vi "Analysis.vi"() -> ()   [LabVIEW 2015, in "SubVIs.lvlib"]
uses:
  SubVIs.lvlib
panel:
  out "SPL":dynamicdata(graph)
  out "Audio":dynamicdata(graph)
  out "Pressure":dynamicdata(graph)
  out "Flow":dynamicdata(graph)
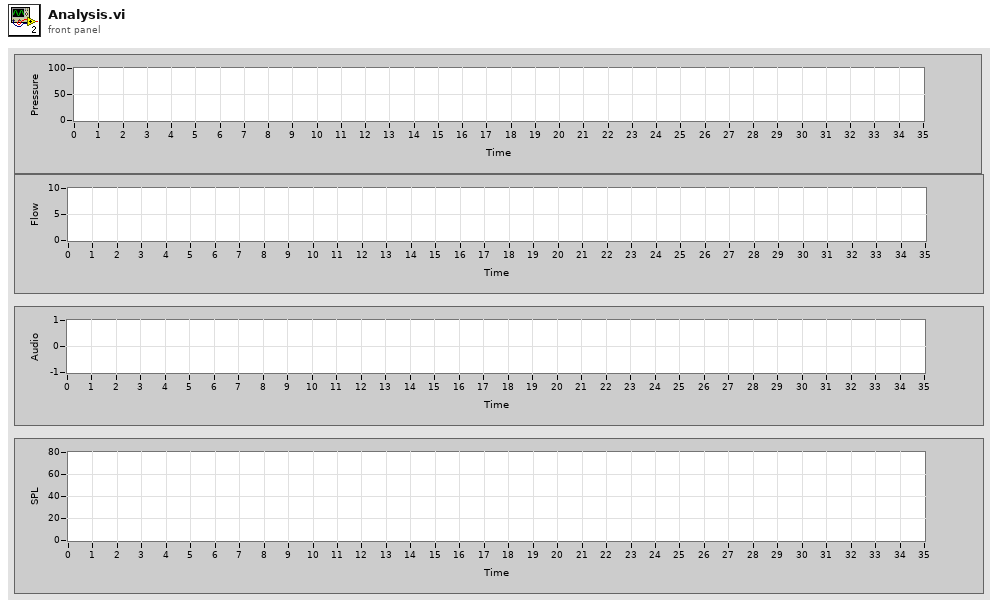
[diagram p1: front panel]
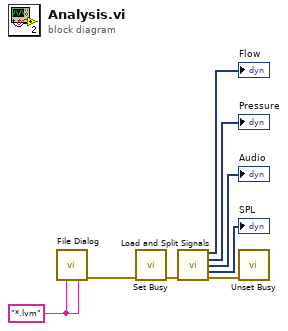
[diagram p0: block diagram]
diagram:
  w4 = "*.lvm" ("pattern (all files)")
  n1 = call "File Dialog"("pattern (all files)"=w4, "pattern label"=w4) -> ("error out"=w3:errorcluster)  [unwired: 10 in, 3 out]
  n2 = call <vilib>:"Set Busy.vi"("error in (no error)"=w3) -> ("error out"=w2:errorcluster)  [unwired: 9 in, 1 out]
  n3 = call "Load and Split Signals.vi"("Error In"=w2) -> ("Flow"=→"Flow":dynamicdata, "Pressure"=→"Pressure":dynamicdata, "Audio"=→"Audio":dynamicdata, "SPL"=→"SPL":dynamicdata, "Error Out"=w1:errorcluster)  [unwired: 8 in, 2 out]
  n4 = call <vilib>:"Unset Busy.vi"("error in (no error)"=w1) -> ()  [unwired: 10 in, 1 out]
